vi "Convex Hull 2D (GiftWrap) example.vi"(1 "Points":sgl[][](array[numeric])=[[0.0, 0.0, 0.0], [10.0, 0.0, 0.0], [10.0, 10.0, 0.0], [0.0, 10.0, 0.0], [50.0, 50.0, 0.0], [60.0, 50.0, 0.0], [60.0, 60.0, 0.0], [50.0, 60.0, 0.0]]) -> (0 "Convex Hull lines":T1[](array[typedef]))   [LabVIEW 2014]
uses:
  Typedefs/Edge.ctl
  Subroutines/Cross product 3D.vi
  Subroutines/Unit vector.vi
panel:
  out "Convex Hull vertices":sgl[][](array[numeric])
  in  "Random start pts":bool=TRUE
  in  "Npts random":i32=32
  out "Visualisation":cluster{sgl[], sgl[]}[](graph)
  # "PN 17/03/2015"
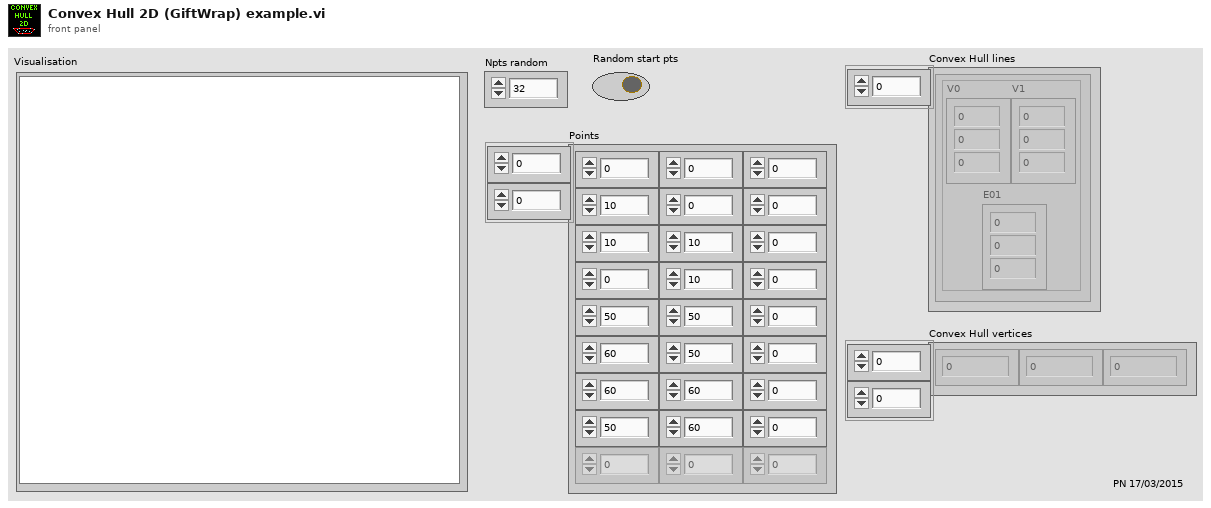
[diagram p1: front panel]
types:
  T1 = typedef "Edge.ctl" = cluster{"V0":sgl[], "V1":sgl[], "E01":sgl[]}
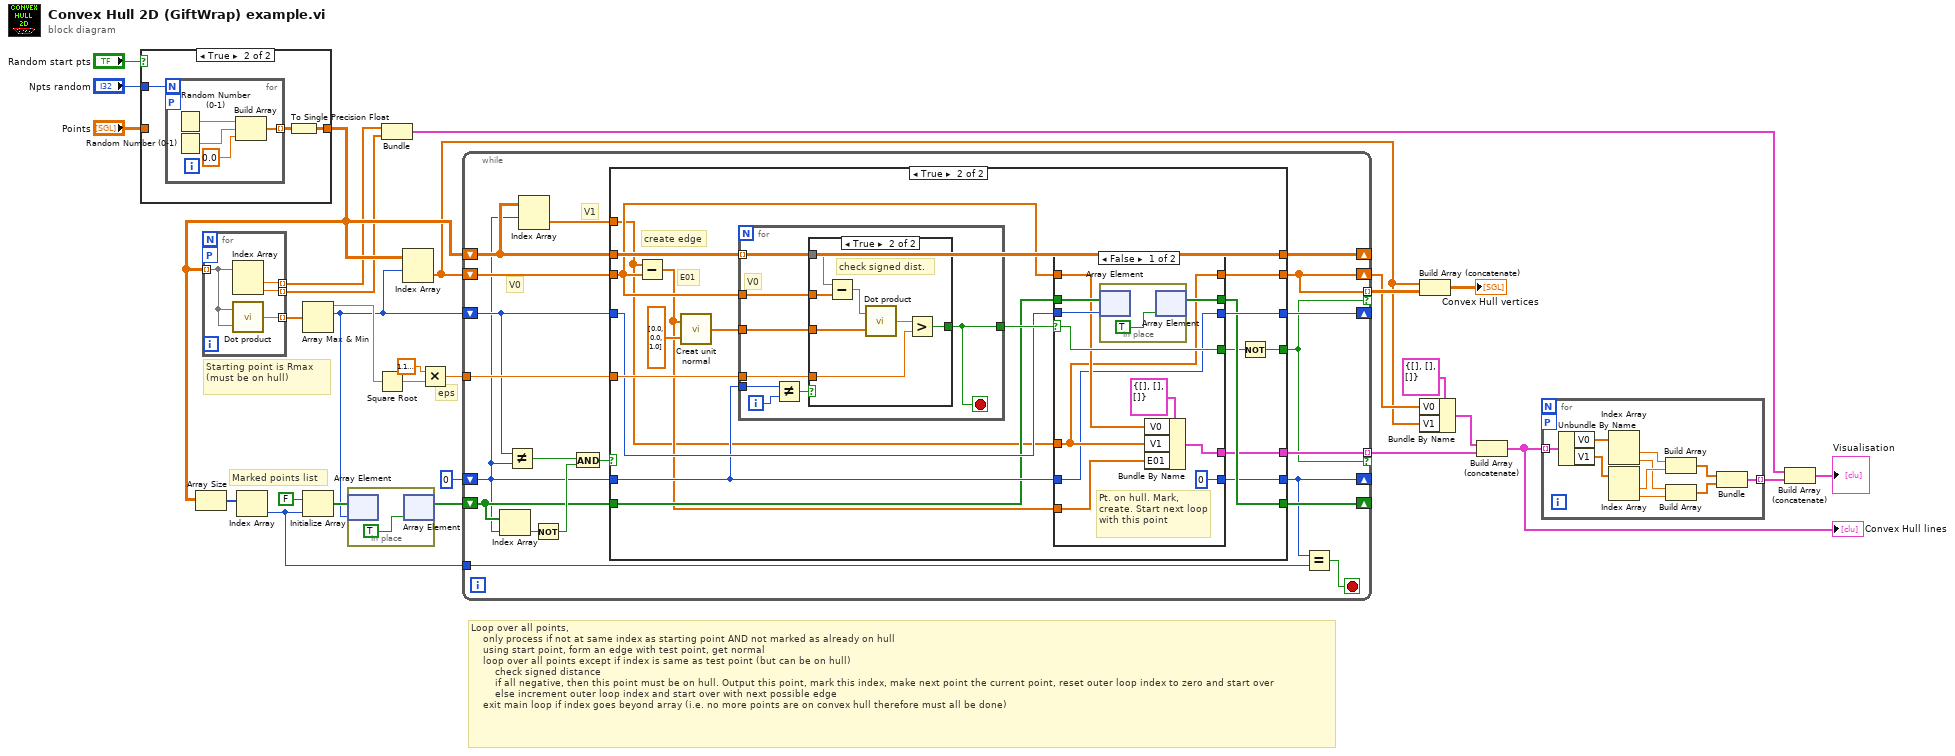
[diagram p0: block diagram]
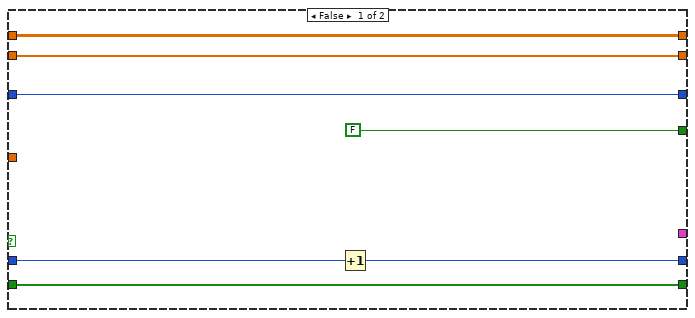
[diagram p2: hidden frame]
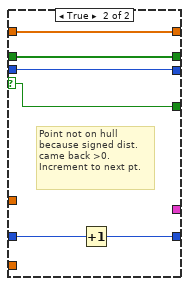
[diagram p3: hidden frame]
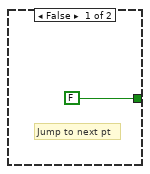
[diagram p4: hidden frame]
diagram:
  # "Loop over all points,\n    only process if not at same index as starting point AND not marked as already on hull\n    using start point, form an edge with test point, get normal\n    loop over all points except if index is same as test point (but can be on hull)\n        check signed distance\n        if all negative, then this point must be on hull. Output this point, mark this index, make next point the current point, reset outer loop index to zero and start over\n        else increment outer loop index and start over with next possible edge\n    exit main loop if index goes beyond array (i.e. no more points are on convex hull therefore must all be done)"
  # "Marked points list"
  # "eps"
  # "Starting point is Rmax (must be on hull)"
  n1 = case shown="True" "Random start pts" {
    tunnel: "Npts random" -> [_ w32]
    tunnel: "Points" -> [w30 _]
    tunnel: [w30 w31] -> w16
    frame False {
    }
    frame True {
      n2 = for {
        N: w32 -> [_]
        tunnel: [w34] -> w33 mode=indexing
        workers-P: _ -> [_]
        n3 = Random Number (0-1)() -> (number: 0 to 1=w37:dbl)
        n4 = Random Number (0-1)() -> (number: 0 to 1=w36:dbl)
        n5 = Build Array(w37, w36, 0.0 ("element")) -> (w34:dbl[])
      }
      n6 = To Single Precision Float(number=w33) -> (single precision float=w31:sgl[][])
    }
  }
  n7 = Array Size(array=w16) -> (size(s)=w17:i32[])
  n8 = for {
    tunnel: w16 -> [w39] mode=indexing
    tunnel: [w41] -> w12 mode=indexing
    tunnel: [w40] -> w11 mode=indexing
    tunnel: [w38] -> w24 mode=indexing
    workers-P: _ -> [_]
    n9 = Index Array(array=w39) -> (element #1=w41:sgl, element #2=w40:sgl)  [unwired: 2 in]
    n10 = call "Dot product.vi"("B"=w39, "A"=w39) -> ("A . B"=w38:sgl)
  }
  n11 = Index Array(array=w17) -> (element=w14:i32)  [unwired: 1 in]
  n12 = Array Max & Min(array=w24) -> (max value=w21:sgl, max index (indices)=w2:i32)  [unwired: 2 out]
  n13 = Initialize Array(FALSE, w14) -> (w3:bool[])
  n14 = in-place {
    n15 = in-place-array #1(w3, w2) -> ()  [unwired: 1 out]
    n16 = in-place-array #1(TRUE) -> (w1:bool[])  [unwired: 1 out]
  }
  n17 = Square Root(x=w21) -> (sqrt(x)=w20:sgl)
  n18 = Bundle(w12, w11) -> (w23:cluster{sgl[], sgl[]})  [unwired: 1 in]
  n19 = Index Array(array=w16, index (row)=w2) -> (element=w5:sgl[])  [unwired: 1 in]
  n20 = Multiply(x=sgl 1.1920929e-07, y=w20) -> (x*y=w19:sgl)
  n21 = while {
    shift-right: [w57] -> _
    shift-left: w16 -> [w52]
    shift-right: [w44] -> w6
    shift-left: w5 -> [w62]
    tunnel: w19 -> [w61]
    shift-right: [w59] -> _
    shift-left: w2 -> [w60]
    shift-right: [w58] -> _
    shift-left: w1 -> [w50]
    tunnel: [w53] -> w8 mode=indexing if=w43
    shift-right: [w46] -> _
    shift-left: 0 -> [w49]
    tunnel: w14 -> [w45]
    tunnel: [w44] -> w13 mode=indexing if=w43
    stop <- w47 stop-if-true
    # "V1"
    # "V0"
    n22 = Index Array(array=w50, index=w49) -> (element=w48:bool)
    n23 = Not Equal?(x=w60, y=w49) -> (x != y?=w56:bool)
    n24 = Index Array(array=w52, index (row)=w49) -> (element=w51:sgl[])  [unwired: 1 in]
    n25 = Not(x=w48) -> (.not. x?=w55:bool)
    n26 = And(x=w56, y=w55) -> (x .and. y?=w54:bool)
    n27 = case shown="True" w54 {
      tunnel: w49 -> [w64 w82]
      tunnel: w51 -> [_ w70]
      tunnel: w62 -> [w69 w77]
      tunnel: w61 -> [_ w86]
      tunnel: w52 -> [w66 w78]
      tunnel: w60 -> [w68 w84]
      tunnel: [w68 w83] -> w59
      tunnel: [w69 w81] -> w44
      tunnel: w50 -> [w67 w80]
      tunnel: [w67 w79] -> w58
      tunnel: [w66 w78] -> w57
      tunnel: [_ w76] -> w53
      tunnel: [FALSE w74] -> w43
      tunnel: [w63 w71] -> w46
      frame False {
        n28 = Increment(x=w64) -> (x+1=w63:i32)
      }
      frame True {
        # "E01"
        # "create edge"
        n29 = Subtract(x=w70, y=w77) -> (x-y=w72:sgl[])
        n30 = call "Creat unit normal.vi"("E2"=sgl[] [0.0, 0.0, 1.0] ("B"), "E1"=w72) -> ("n^ = (E1 x E2) / ||E1 x E2||"=w73:sgl[])
        n31 = for {
          tunnel: w73 -> [w110]
          tunnel: w78 -> [w109] mode=indexing
          tunnel: w82 -> [w112]
          tunnel: w77 -> [w108]
          tunnel: w86 -> [w107]
          tunnel: [w106] -> w85
          i -> [w113]
          stop <- w106 stop-if-true
          # "V0"
          n32 = Not Equal?(x=w112, y=w113) -> (x != y?=w111:bool)
          n33 = case shown="True" w111 {
            tunnel: w110 -> [_ w121]
            tunnel: w109 -> [_ w120]
            tunnel: w108 -> [_ w119]
            tunnel: [FALSE w115] -> w106
            tunnel: w107 -> [_ w116]
            frame False {
              # "Jump to next pt"
            }
            frame True {
              # "check signed dist."
              n34 = Subtract(x=w120, y=w119) -> (x-y=w118:sgl[])
              n35 = call "Dot product.vi"("B"=w121, "A"=w118) -> ("A . B"=w117:sgl)
              n36 = Greater?(x=w117, y=w116) -> (0:w115:bool)
            }
          }
        }
        n37 = case shown="False" w85 {
          selector: w85 -> [w93 w102]
          tunnel: w84 -> [w97 w104]
          tunnel: [w88 w104] -> w83
          tunnel: w82 -> [w88 w101]
          tunnel: w70 -> [w89 _]
          tunnel: [w89 w105] -> w81
          tunnel: w80 -> [w98 w103]
          tunnel: w77 -> [w92 w105]
          tunnel: [w96 w103] -> w79
          tunnel: [w94 _] -> w76
          tunnel: [w93 w102] -> w75
          tunnel: w72 -> [w91 _]
          tunnel: [0 w100] -> w71
          frame False {
            # "Pt. on hull. Mark, create. Start next loop with this point"
            n38 = in-place {
              n39 = in-place-array #2(w98, w97) -> ()  [unwired: 1 out]
              n40 = in-place-array #2(TRUE) -> (w96:bool[])  [unwired: 1 out]
            }
            n41 = Bundle By Name(cluster=T1 {"V0"=[], "V1"=[], "E01"=[]} ("Edge"), "V0"=w92, "V1"=w89, "E01"=w91) -> (w94:T1)
          }
          frame True {
            # "Point not on hull because signed dist. came back >0.\nIncrement to next pt."
            n42 = Increment(x=w101) -> (x+1=w100:i32)
          }
        }
        n43 = Not(x=w75) -> (.not. x?=w74:bool)
      }
    }
    n44 = Equal?(x=w46, y=w45) -> (x = y?=w47:bool)
  }
  n45 = Build Array (concatenate)(w5, w13) -> (→"Convex Hull vertices":sgl[][])
  n46 = Bundle By Name(cluster=T1 {"V0"=[], "V1"=[], "E01"=[]} ("Edge"), "V0"=w6, "V1"=w5) -> (w4:T1)
  n47 = Build Array (concatenate)(w4, w8) -> (w7:T1[])
  "Convex Hull lines" <- w7
  n48 = for {
    tunnel: [w123] -> w28 mode=indexing
    workers-P: _ -> [_]
    tunnel: w7 -> [w122] mode=indexing
    n49 = Unbundle By Name(w122) -> ("V0"=w125:sgl[], "V1"=w124:sgl[])
    n50 = Index Array(array=w125) -> (element #1=w131:sgl, element #2=w128:sgl)  [unwired: 2 in]
    n51 = Index Array(array=w124) -> (element #1=w129:sgl, element #2=w127:sgl)  [unwired: 2 in]
    n52 = Build Array(w131, w129) -> (w130:sgl[])
    n53 = Build Array(w128, w127) -> (w126:sgl[])
    n54 = Bundle(w130, w126) -> (w123:cluster{sgl[], sgl[]})  [unwired: 1 in]
  }
  n55 = Build Array (concatenate)(w23, w28) -> (→"Visualisation":cluster{sgl[], sgl[]}[])
